vi "Create Constant.vi"(0 "Terminal in":refnum<vi>, 11 "error in (no error)":errorcluster) -> (4 "Terminal out":refnum<vi>, 6 "Create Constant":refnum<vi>, 15 "error out":errorcluster)   [LabVIEW 2021, in "Converter.lvlib"]
uses:
  Converter.lvlib
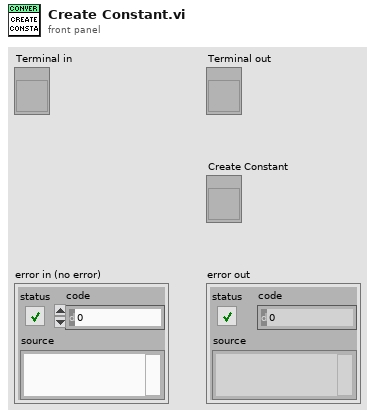
[diagram p1: front panel]
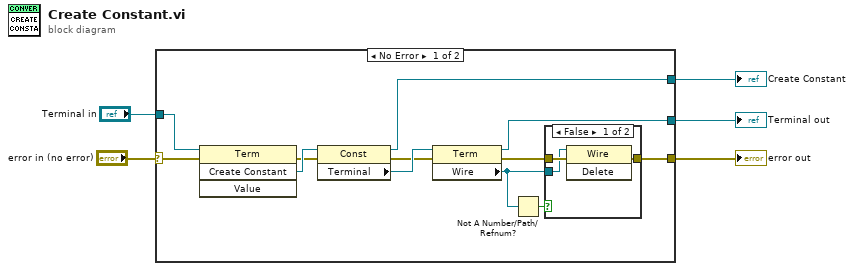
[diagram p0: block diagram]
diagram:
  n1 = case shown="No Error" "error in (no error)" {
    selector: "error in (no error)" -> [w13 w22]
    tunnel: "Terminal in" -> [w15 _]
    tunnel: [w8 w22] -> w3
    tunnel: [w7 _] -> w2
    tunnel: [w6 _] -> w1
    frame No Error {
      n2 = invoke class="Term" method="Create Constant"(reference=w15, error in=w13) -> (error out=w12:errorcluster, "Create Constant"=w14:refnum<vi>)  [unwired: 2 in, 2 out]
      n3 = property class="Const"(reference=w14, error in=w12) -> (reference out=w6:refnum<vi>, error out=w10:errorcluster, "Terminal"=w11:refnum<vi>)
      n4 = property class="Term"(reference=w11, error in=w10) -> (reference out=w7:refnum<vi>, error out=w9:errorcluster, "Wire"=w16:refnum<vi>)
      n5 = Not A Number/Path/Refnum?(number/path/refnum=w16) -> (NaN/Path/Refnum?=w17:bool)
      n6 = case shown="False" w17 {
        tunnel: [w20 w21] -> w8
        tunnel: w9 -> [w19 w21]
        tunnel: w16 -> [w18 _]
        frame False {
          n7 = invoke class="Wire" method="Delete"(reference=w18, error in=w19) -> (error out=w20:errorcluster)  [unwired: 1 in, 2 out]
        }
        frame True {
        }
      }
    }
    frame Error {
    }
  }
  "error out" <- w3
  "Terminal out" <- w2
  "Create Constant" <- w1
